vi "tcpvi name.vi"() -> (3 "tcpvi name":string)   [LabVIEW 2013]
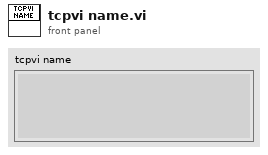
[diagram p1: front panel]
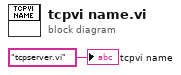
[diagram p0: block diagram]
diagram:
  "tcpvi name" <- "tcpserver.vi" ("name or relative path")
